vi "IncrementIndex.vi"(8 "Increment?":bool, 11 "IndexIn":i32) -> (3 "IndexOut":i32)   [LabVIEW 2017]
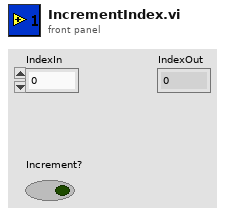
[diagram p1: front panel]
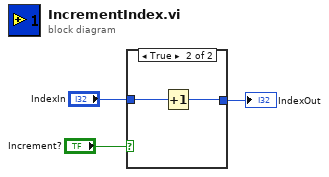
[diagram p0: block diagram]
diagram:
  n1 = case shown="True" "Increment?" {
    tunnel: "IndexIn" -> [w4 w6]
    tunnel: [w4 w5] -> w1
    frame False {
    }
    frame True {
      n2 = Increment(x=w6) -> (x+1=w5:i32)
    }
  }
  "IndexOut" <- w1
